vi "FourierTransform.vi"() -> ()   [LabVIEW 2013]
panel:
  out "Fourier transform 2":cluster{"X":dbl[], "Y":dbl[]}[](graph)
  out "Fourier transform":cluster{dbl[], dbl[]}(graph)
  in  "NT":dbl caption="Numero de ciclos (N)" format="%#_13g"
  in  "Numero de harmonicas(n)":dbl
  in  "Precisao temporal (dt)":dbl
  in  "Periodo (T)":dbl
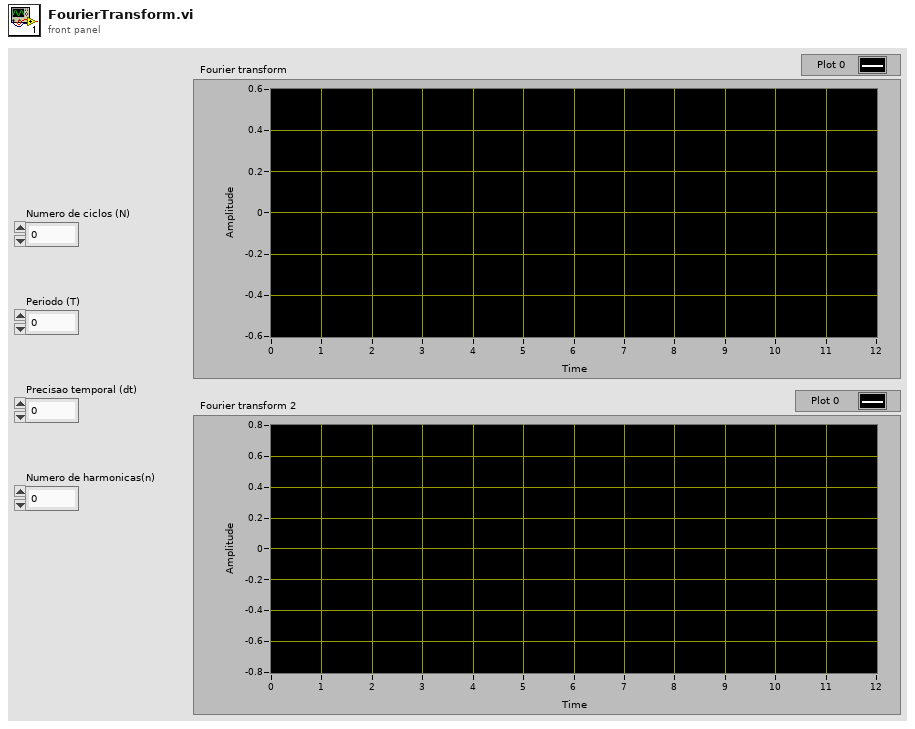
[diagram p1: front panel]
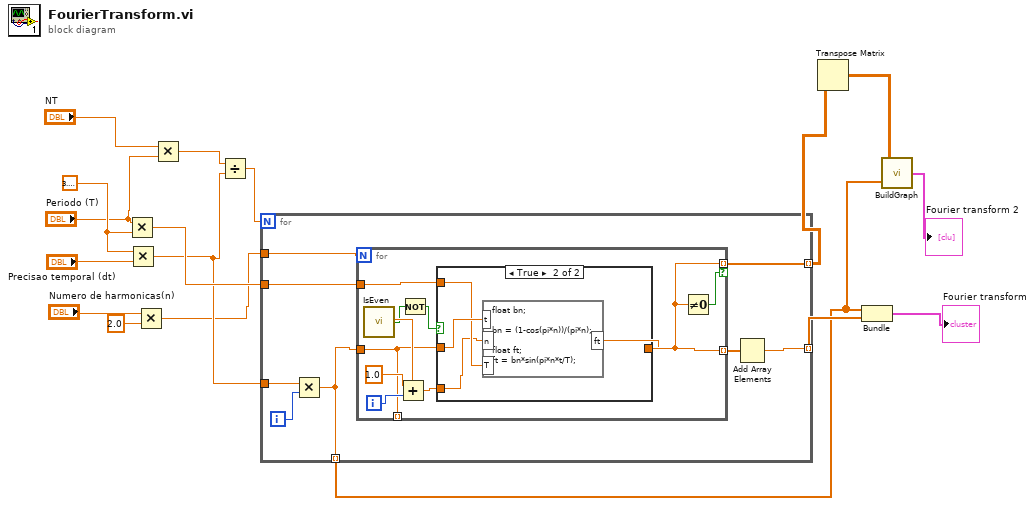
[diagram p0: block diagram]
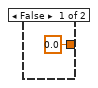
[diagram p2: hidden frame]
diagram:
  w17 = 3.141592653589793
  n1 = Multiply(x="Periodo (T)", y=w17) -> (x*y=w14:dbl)
  n2 = Multiply(x=w17, y="Precisao temporal (dt)") -> (x*y=w11:dbl)
  n3 = Multiply(x="Numero de harmonicas(n)", y=2.0) -> (x*y=w5:dbl)
  n4 = Multiply(x="NT", y="Periodo (T)") -> (x*y=w12:dbl)
  n5 = Divide(x=w12, y=w11) -> (x/y=w10:dbl)
  n6 = for {
    N: w10 -> [_]
    tunnel: w11 -> [w24]
    tunnel: w5 -> [w23]
    tunnel: w14 -> [w22]
    tunnel: [w20] -> w9 mode=indexing
    tunnel: [w19] -> w4 mode=indexing
    tunnel: [w18] -> w2 mode=indexing
    i -> [w25]
    n7 = Multiply(x=w24, y=w25) -> (x*y=w19:dbl)
    n8 = for {
      N: w23 -> [_]
      tunnel: [w26] -> w21 mode=indexing
      tunnel: w19 -> [w30]
      tunnel: w22 -> [w31]
      tunnel: [w30] -> _ mode=indexing
      tunnel: [w26] -> w18 mode=indexing if=w27
      i -> [w34]
      n9 = Add(x=1.0, y=w34) -> (x+y=w32:dbl)
      n10 = call "IsEven.vi"("Numeric"=w32) -> ("Boolean"=w29:bool)
      n11 = Not(x=w29) -> (.not. x?=w28:bool)
      n12 = case shown="True" w28 {
        tunnel: [0.0 w37] -> w26
        tunnel: w32 -> [_ w36]
        tunnel: w30 -> [_ w39]
        tunnel: w31 -> [_ w38]
        frame False {
        }
        frame True {
          n13 = formula code="float bn;\n\nbn = (1-cos(pi*n))/(pi*n);\n\nfloat ft;\nft = bn*sin(pi*n*t/T);"("t"=w39, "n"=w36, "T"=w38) -> ("ft"=w37:dbl)
        }
      }
      n14 = Not Equal To 0?(x=w26) -> (x != 0?=w27:bool)
    }
    n15 = Add Array Elements(numeric array=w21) -> (sum=w20:dbl)
  }
  n16 = Transpose Matrix(1:w2) -> (0:w1:dbl[][])
  n17 = Bundle(w4, w9) -> (→"Fourier transform":cluster{dbl[], dbl[]})  [unwired: 1 in]
  n18 = call "BuildGraph.vi"("X"=w4, "Y"=w1) -> ("Graph"=→"Fourier transform 2":cluster{"X":dbl[], "Y":dbl[]}[])
